vi "Numeric_bins_test.vi"(1 "Tolerance":dbl=0.02 format="%.3f", 2 "Values":dbl[](array[numeric])=[1.9842, 1.9891, 1.9908, 1.9921, 1.99931, 1.9971, 1.9981, 1.9985, 1.999, 1.9992, 2.0001, 2.0024, 2.0041, 2.007, 2.0072, 2.009, 2.0115, 2.0199, 2.0244] format="%.4f") -> (0 "Bin Centres":dbl[](array[numeric])=[1.996462307692308, 2.0131666666666668] format="%.4f")   [LabVIEW 2010]
panel:
  out "Bin Number":i32[](array[numeric])
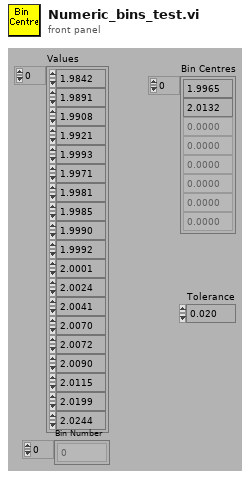
[diagram p1: front panel]
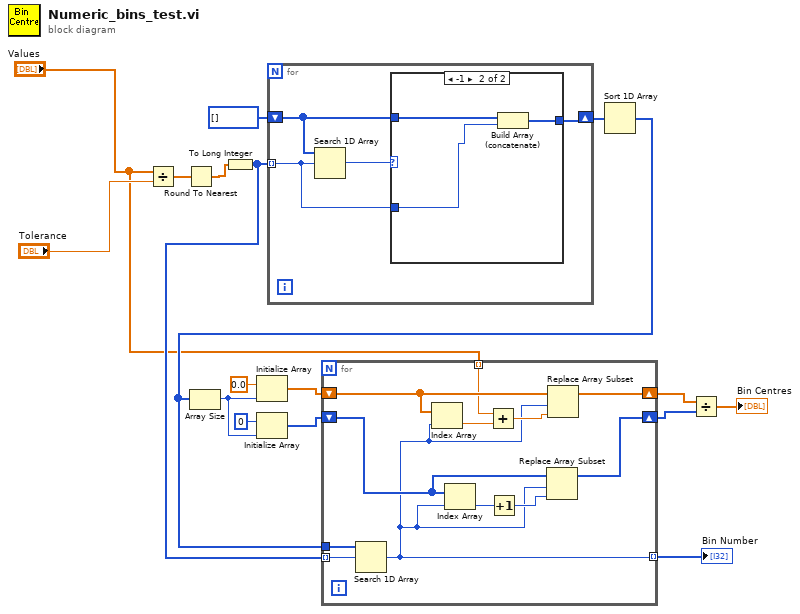
[diagram p0: block diagram]
diagram:
  n1 = Divide(x="Values", y="Tolerance") -> (x/y=w17:dbl[])
  n2 = Round To Nearest(number=w17) -> (nearest integer value=w16:dbl[])
  n3 = To Long Integer(number=w16) -> (32bit integer=w12:i32[])
  n4 = for {
    shift-right: [w19] -> w13
    shift-left: i32[] [] -> [w18]
    tunnel: w12 -> [w20] mode=indexing
    n5 = Search 1D Array(1D array=w18, element=w20) -> (index of element=w21:i32)  [unwired: 1 in]
    n6 = case shown="-1" w21 {
      tunnel: w18 -> [w22 w25]
      tunnel: w20 -> [_ w24]
      tunnel: [w22 w23] -> w19
      frame 0, Default {
      }
      frame -1 {
        n7 = Build Array (concatenate)(w25, w24) -> (w23:i32[])
      }
    }
  }
  n8 = Sort 1D Array(array=w13) -> (sorted array=w11:i32[])
  n9 = Array Size(array=w11) -> (size(s)=w7:i32)
  n10 = Initialize Array(0.0 ("element"), w7) -> (w9:dbl[])
  n11 = Initialize Array(0 ("element"), w7) -> (w6:i32[])
  n12 = for {
    tunnel: w11 -> [w37]
    tunnel: w12 -> [w36] mode=indexing
    shift-right: [w34] -> w4
    shift-left: w9 -> [w35]
    shift-right: [w33] -> w3
    shift-left: w6 -> [w32]
    tunnel: "Values" -> [w27] mode=indexing
    tunnel: [w26] -> w1 mode=indexing
    n13 = Search 1D Array(1D array=w37, element=w36) -> (index of element=w26:i32)  [unwired: 1 in]
    n14 = Index Array(array=w35, index=w26) -> (element=w29:dbl)
    n15 = Index Array(array=w32, index=w26) -> (element=w31:i32)
    n16 = Add(x=w27, y=w29) -> (x+y=w28:dbl)
    n17 = Increment(x=w31) -> (x+1=w30:i32)
    n18 = Replace Array Subset(array=w32, new element=w30, index=w26) -> (w33:i32[])
    n19 = Replace Array Subset(array=w35, new element=w28, index=w26) -> (w34:dbl[])
  }
  "Bin Number" <- w1
  n20 = Divide(x=w4, y=w3) -> (x/y=→"Bin Centres":dbl[])
